vi "n_abs.vi"(2 "n_excess":dbl, 3 "rho_ads":dbl, 4 "Pf":dbl, 5 "z":dbl, 6 "T":dbl, 7 "MW":dbl) -> (0 "n_abs":dbl, 1 "rho_bulk":dbl)   [LabVIEW 2016]
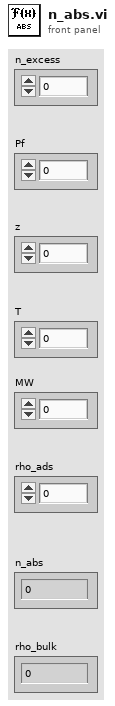
[diagram p1: front panel]
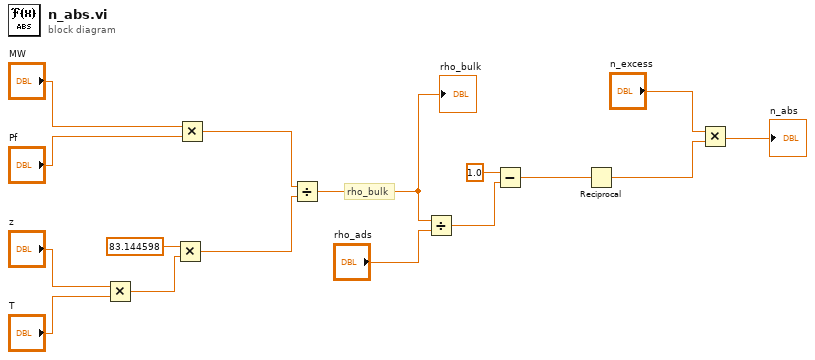
[diagram p0: block diagram]
diagram:
  # "rho_bulk"
  n1 = Multiply(x="z", y="T") -> (x*y=w12:dbl)
  n2 = Multiply(x=83.144598, y=w12) -> (x*y=w9:dbl)
  n3 = Multiply(x="MW", y="Pf") -> (x*y=w10:dbl)
  n4 = Divide(x=w10, y=w9) -> (x/y=w1:dbl)
  "rho_bulk" <- w1
  n5 = Divide(x=w1, y="rho_ads") -> (x/y=w7:dbl)
  n6 = Subtract(x=1.0, y=w7) -> (x-y=w5:dbl)
  n7 = Reciprocal(x=w5) -> (1/x=w3:dbl)
  n8 = Multiply(x="n_excess", y=w3) -> (x*y=→"n_abs":dbl)
